vi "GetText.vi"(8 "error in":errorcluster, 11 "node in":refnum<class "RunTimeObjectsSection.lvclass">) -> (0 "error out":errorcluster, 1 "additional text":string, 2 "text":string, 3 "node out":refnum<class "RunTimeObjectsSection.lvclass">, 4 "glyph":string)   [LabVIEW 2015, in "RunTimeObjectsSection.lvclass"]
doc: "Returns the text representation of the node used for the tree control."
uses:
  RunTimeObjectsSection.lvclass
  RunTimeObjectsSection.lvclass/RunTimeObjectsSection.ctl
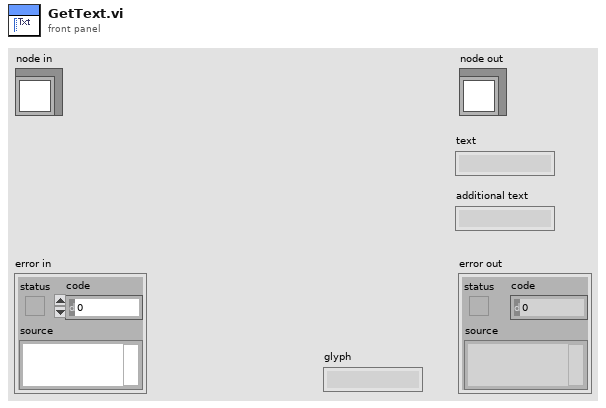
[diagram p1: front panel]
types:
  T1 = typedef "RunTimeObjectTypes.ctl" = enum16{"ActionVIs", "ButtonList", "RunTimeMenu"}
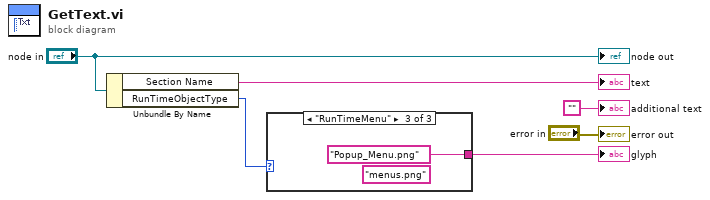
[diagram p0: block diagram]
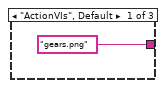
[diagram p2: hidden frame]
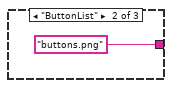
[diagram p3: hidden frame]
diagram:
  n1 = Unbundle By Name("node in") -> ("Section Name"=→"text":string, "RunTimeObjectType"=w2:T1)
  n2 = case shown="\"RunTimeMenu\"" w2 {
    tunnel: ["gears.png" ("glyph") "buttons.png" ("glyph") "Popup_Menu.png" ("glyph")] -> w1
    frame "ActionVIs", Default {
    }
    frame "ButtonList" {
    }
    frame "RunTimeMenu" {
      (unwired) "menus.png" ("glyph")
    }
  }
  "glyph" <- w1
  "error out" <- "error in"
  "node out" <- "node in"
  "additional text" <- ""
